vi "Change State.vi"(8 "error in (no error)":errorcluster, 10 "State Types":T1, 11 "Model in":refnum<class "Model.lvclass">) -> (0 "error out":errorcluster, 3 "Model out":refnum<class "Model.lvclass">)   [LabVIEW 2015, in "Model.lvclass"]
uses:
  Model.lvclass
  Typedefs/StateTypes.ctl
  Model.lvclass/Model.ctl
  User Events/User Events.lvclass/User Events.ctl
  User Events/User Events.lvclass
  Typedefs/FAMT Typedefs.lvlib
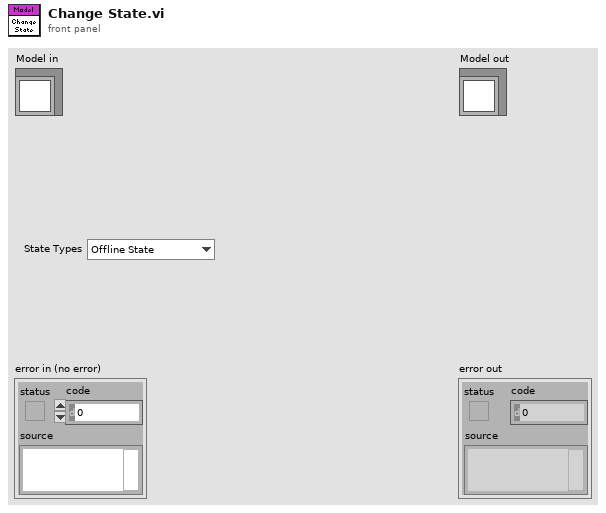
[diagram p1: front panel]
types:
  T1 = typedef "FAMT Typedefs.lvlib/StateTypes.ctl" = enum16{"Offline State", "Fault State", "Standby State", "Disabled State", "Enabled State", "Wait For User Input State", "Perform Scan State"}
  T2 = typedef "FAMT Typedefs.lvlib/Publish Data Events.ctl" = cluster{"State":refnum<user-event>, "ErrorCode":refnum<user-event>, "FC1 ILC Outputs":refnum<user-event>, "LogPath":refnum<user-event>, "FC1 ILC Inputs":refnum<user-event>, "Scan Progress":refnum<user-event>, "FC2 ILC Outputs":refnum<user-event>, "FC2 ILC Inputs":refnum<user-event>}
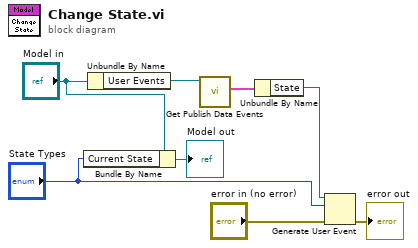
[diagram p0: block diagram]
diagram:
  n1 = Bundle By Name(cluster="Model in", "Current State"="State Types") -> (→"Model out":refnum<class "Model.lvclass">)
  n2 = Unbundle By Name("Model in") -> ("User Events"=w5:refnum<class "User Events.lvclass">)
  n3 = call "Get Publish Data Events.vi"("UserEvents in"=w5) -> ("Publish Data Events"=w4:T2)  [unwired: 9 in, 1 out]
  n4 = Unbundle By Name(w4) -> ("State"=w3:refnum<user-event>)
  n5 = Generate User Event(user event=w3, event data cluster="State Types", error in="error in (no error)") -> (error out=→"error out":errorcluster)  [unwired: 1 in, 1 out]
